vi "Single Measure Gate Frequency Query.vi"(8 "error in":errorcluster, 11 "Instrument Handle In":i32) -> (0 "error out":errorcluster, 1 "Gate Stop Freq":dbl, 2 "Gate Start Freq":dbl, 3 "Instrument Handle Out":i32)   [LabVIEW 8.6, in "ZTScopeM.lvlib"]
doc: "Query the measurement gate start and stop positions based on frequency."
uses:
  ZTScopeM.lvlib
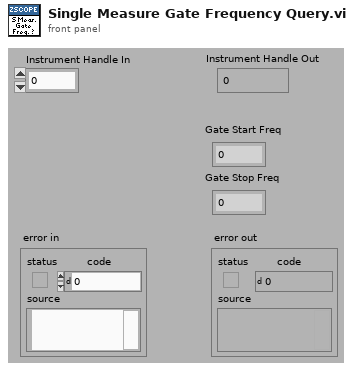
[diagram p1: front panel]
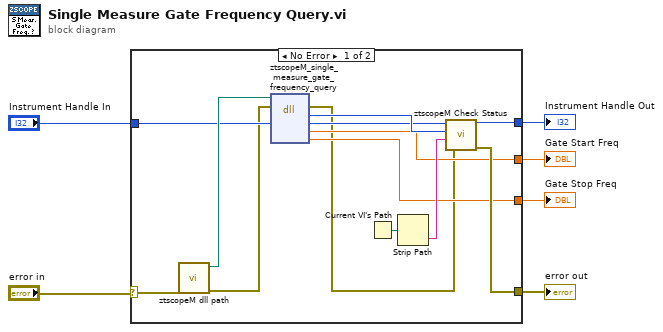
[diagram p0: block diagram]
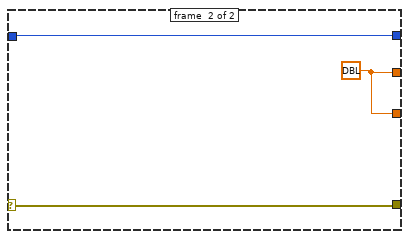
[diagram p2: hidden frame]
diagram:
  n1 = case shown="No Error" "error in" {
    selector: "error in" -> [w11 w22]
    tunnel: [w14 w22] -> w5
    tunnel: [w15 w20] -> w4
    tunnel: [w13 w21] -> w3
    tunnel: [w12 w21] -> w2
    tunnel: "Instrument Handle In" -> [w9 w20]
    frame #0 {
      n2 = call "ztscopeM dll path.vi"("error in (no error)"=w11) -> ("error out"=w8:errorcluster, "<instrument>.dll path"=w10:path)  [unwired: 9 in]
      n3 = dll-call lib="C:/Program Files (x86)/National Instruments/LabVIEW 2013/instr.lib/ztscopem/ztscopeM.dll" fn="ztscopeM_single_measure_gate_frequency_query"(path in=w10, error in=w8, "instrumentHandle"=w9) -> (error out=w7:errorcluster, w19:i32, "instrumentHandle"=w18:i32, "gateStart"=w13:dbl, "gateStop"=w12:dbl)  [unwired: 1 in, 3 out]
      n4 = Current VI's Path() -> (path=w17:path)
      n5 = Strip Path(path=w17) -> (name=w16:string)  [unwired: 1 out]
      n6 = call "ztscopeM Check Status.vi"("error in"=w7, "name of VI"=w16, "status (return code)"=w19, "instrument handle in"=w18) -> ("error out"=w14:errorcluster, "instrument handle out"=w15:i32)  [unwired: 2 out]
    }
    frame #1 {
      w21 = dbl ? ("instrumentHandle")
    }
  }
  "Instrument Handle Out" <- w4
  "error out" <- w5
  "Gate Start Freq" <- w3
  "Gate Stop Freq" <- w2
